vi "1.3子程序.vi"() -> (0 "0-10随机数并与10相乘":dbl)   [LabVIEW 2016]
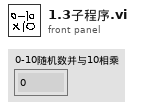
[diagram p1: front panel]
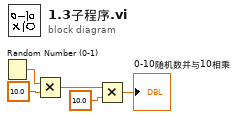
[diagram p0: block diagram]
diagram:
  n1 = Random Number (0-1)() -> (number: 0 to 1=w4:dbl)
  n2 = Multiply(x=w4, y=10.0) -> (x*y=w3:dbl)
  n3 = Multiply(x=w3, y=10.0) -> (x*y=→"0-10随机数并与10相乘":dbl)
